vi "Test Process Error in Process Loop Log Error Message.vi"(8 "error in (no error)":errorcluster, 11 "Test Case In":refnum<class "Logger Test.lvclass">) -> (0 "error out":errorcluster, 3 "Test Case Out":refnum<class "Logger Test.lvclass">)   [LabVIEW 2020, in "Logger Test.lvclass"]
uses:
  Logger Test.lvclass
  C:/Program Files (x86)/National Instruments/LabVIEW 2020/vi.lib/Astemes/LUnit/Test Case.lvclass
  source/Framework Test Suite/Mock Log Handler/Mock Log Handler.lvclass
  C:/Git/astemes-triarc-framework/source/Framework/Logging/Logging.lvclass
  source/Framework Test Suite/Mock Process/Mock Process.lvclass
  C:/Git/astemes-triarc-framework/source/Framework/Process/Process.lvclass
  source/Framework/Process/Process.lvclass/Process.ctl
  <vilib>/Astemes/LUnit/Test Case.lvclass/Test Case.ctl
  9649ef94-fae4-4853-88e7-0393d3ac6ac8.vi
  source/Framework/Process/Public/Lifecycle/Get Lifecycle State.vi
  source/Framework/Process/Protected/Messaging/Send Message.vi
  source/Framework/Process/Private/SubVIs/Wait for finish.vi
  source/Framework/Process/Private/SubVIs/Set Lifecycle State.vi
  <vilib>/Astemes/LUnit/Palette/Pass.vi
  <vilib>/Astemes/LUnit/Palette/Fail.vi
  <vilib>/Astemes/LUnit/Compare Variants.vi
  <vilib>/Astemes/LUnit/Describe Comparison.vi
  <vilib>/Astemes/LUnit/Set Assertion Type.vi
  <vilib>/Utility/error.llb/Clear Errors.vi
  source/Framework/Process/Private/SubVIs/Handle Debug Data.vi
  <vilib>/Astemes/LUnit/Add test result.vi
  <vilib>/Astemes/LUnit/Variant to string.vi
  <vilib>/Utility/High Resolution Relative Seconds.vi
  <vilib>/Astemes/LUnit/LUnit Record Assertion Result.vi
  <vilib>/Astemes/LUnit/LUnit Aggregate Assertion Results.vi
  <vilib>/Astemes/LUnit/Method Result/LUnit Merge Status.vi
  <vilib>/Astemes/LUnit/LUnit Concatenate result strings.vi
  <vilib>/Utility/error.llb/Error Cluster From Error Code.vi
  <vilib>/Utility/Data Type/Get Type Information.vi
  <vilib>/Utility/LVClass/Get LV Class Name.vi
  source/Framework/Process/Process.lvclass
  Logger Test.lvclass/Logger Test.ctl
  source/Framework Test Suite/Support/Test Support.lvlib
  C:/Git/astemes-triarc-framework/source/Framework/Base/Base.lvclass
  C:/Git/astemes-triarc-framework/source/Framework/Configuration File/Configuration File.lvclass
  C:/Git/astemes-triarc-framework/source/Framework/Configuration/Configuration.lvclass
  C:/Git/astemes-triarc-framework/source/Framework/Error Handler Interface/Error Handler Interface.lvclass
  C:/Git/astemes-triarc-framework/source/Framework Test Suite/Mock Process/Mock Process.lvclass
  C:/Git/astemes-triarc-framework/source/Framework/Async Handler/Async Handler.lvclass
  C:/Git/astemes-triarc-framework/source/Framework/Helper Loop/Helper Loop.lvclass
  C:/Git/astemes-triarc-framework/source/Framework Test Suite/Mock Log Handler/Mock Log Handler.lvclass
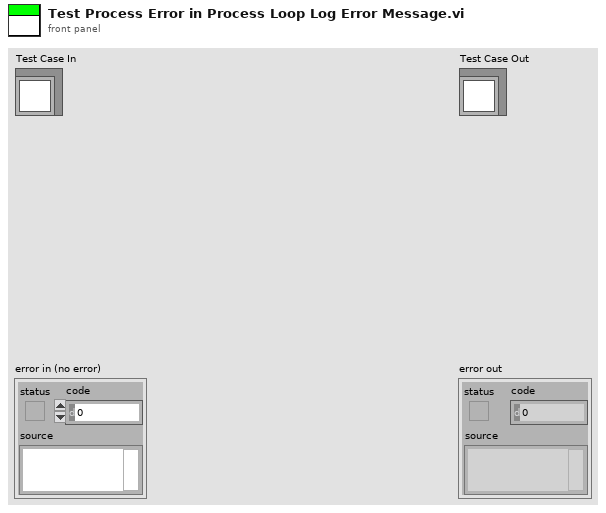
[diagram p1: front panel]
types:
  T1 = typedef "Mock Log Handler.lvclass/Log Entry.ctl" = cluster{"Level":string, "Source":string, "Message":string}
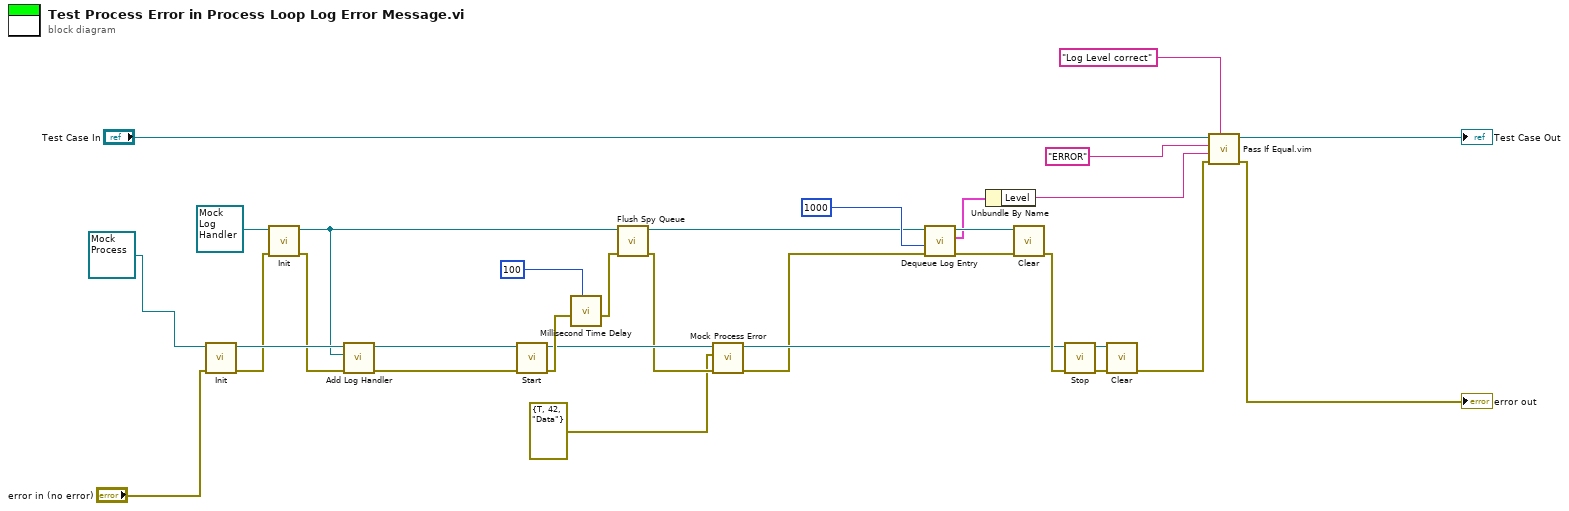
[diagram p0: block diagram]
diagram:
  n1 = call-dynamic "Init.vi"("error in (no error)"="error in (no error)", "Mock Process In"=refnum<class "Mock Process.lvclass"> refnum) -> ("error out"=w26:errorcluster, "Mock Process Out"=w29:refnum<class "Mock Process.lvclass">)  [unwired: 8 in]
  n2 = call-dynamic "Init.vi"("error in (no error)"=w26, "Mock Log Handler In"=refnum<class "Mock Log Handler.lvclass"> refnum ("Mock Log Handler.lvclass")) -> ("error out"=w25:errorcluster, "Mock Log Handler Out"=w13:refnum<class "Mock Log Handler.lvclass">)  [unwired: 8 in]
  n3 = call "Add Log Handler.vi"("error in (no error)"=w25, "Log Handler"=w13, "Process In"=w29) -> ("error out"=w16:errorcluster, "Process Out"=w7:refnum<class "Mock Process.lvclass">)  [unwired: 7 in]
  n4 = call "Start.vi"("error in (no error)"=w16, "Process In"=w7) -> ("error out"=w11:errorcluster, "Process Out"=w5:refnum<class "Mock Process.lvclass">)  [unwired: 7 in, 1 out]
  n5 = call "Millisecond Time Delay.vi"("milliseconds to wait"=u32 100, "error in (no error)"=w11) -> ("error out"=w10:errorcluster)  [unwired: 7 in]
  n6 = call "Flush Spy Queue.vi"("error in (no error)"=w10, "Mock Log Handler in"=w13) -> ("error out"=w3:errorcluster, "Mock Log Handler out"=w12:refnum<class "Mock Log Handler.lvclass">)  [unwired: 7 in, 1 out]
  n7 = call "Mock Process Error.vi"("error in (no error)"=w3, "Mock Error"=errorcluster {"status"=TRUE, "code"=42, "source"="Data"} ("error in (no error)"), "Mock Process in"=w5) -> ("error out"=w2:errorcluster, "Mock Process out"=w4:refnum<class "Mock Process.lvclass">)  [unwired: 7 in]
  n8 = call "Dequeue Log Entry.vi"("error in (no error)"=w2, "timeout in ms (-1)"=1000, "Mock Log Handler in"=w12) -> ("error out"=w23:errorcluster, "Entry"=w20:T1, "Mock Log Handler out"=w24:refnum<class "Mock Log Handler.lvclass">)  [unwired: 5 in, 1 out]
  n9 = Unbundle By Name(w20) -> ("Level"=w19:string)
  n10 = call-dynamic "Clear.vi"("error in (no error)"=w23, "Mock Log Handler In"=w24) -> ("error out"=w21:errorcluster)  [unwired: 9 in]
  n11 = call "Stop.vi"("error in (no error)"=w21, "Process In"=w4) -> ("error out"=w15:errorcluster, "Process Out"=w14:refnum<class "Mock Process.lvclass">)  [unwired: 7 in, 1 out]
  n12 = call-dynamic "Clear.vi"("error in (no error)"=w15, "Mock Process In"=w14) -> ("error out"=w28:errorcluster)  [unwired: 9 in]
  n13 = call "Pass If Equal.vim"("Description"="Log Level correct", "error in (no error)"=w28, "Actual"=w19, "Expected"="ERROR", "LUnit Test Case In"="Test Case In") -> ("error out"=→"error out":errorcluster, "LUnit Test Case Out"=→"Test Case Out":refnum<class "Logger Test.lvclass">)  [unwired: 5 in]
